vi "Init Behavior Lights.vi"() -> (2 "Lights Out":cluster{"Red":bool, "Blue":bool, "Green":bool})   [LabVIEW 2014]
panel:
  # "Flashed Behavior Lights\nRandomly"
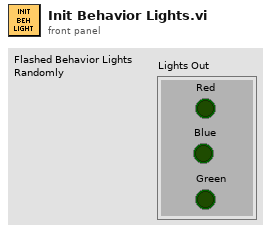
[diagram p1: front panel]
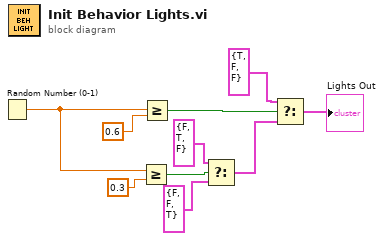
[diagram p0: block diagram]
diagram:
  n1 = Random Number (0-1)() -> (number: 0 to 1=w6:dbl)
  n2 = Greater Or Equal?(x=w6, y=0.3) -> (x >= y?=w7:bool)
  n3 = Greater Or Equal?(x=w6, y=0.6) -> (x >= y?=w9:bool)
  n4 = Select(t=cluster{"Red":bool, "Blue":bool, "Green":bool} {"Red"=FALSE, "Blue"=TRUE, "Green"=FALSE} ("Lights Out"), s=w7, f=cluster{"Red":bool, "Blue":bool, "Green":bool} {"Red"=FALSE, "Blue"=FALSE, "Green"=TRUE} ("Lights Out")) -> (s? t:f=w8:cluster{"Red":bool, "Blue":bool, "Green":bool})
  n5 = Select(t=cluster{"Red":bool, "Blue":bool, "Green":bool} {"Red"=TRUE, "Blue"=FALSE, "Green"=FALSE} ("Lights Out"), s=w9, f=w8) -> (s? t:f=→"Lights Out":cluster{"Red":bool, "Blue":bool, "Green":bool})
